vi "Get Test Values.vi"(8 "error in":errorcluster, 11 "Measurements":waveform(dbl)[](array[waveform])) -> (0 "error out":errorcluster, 1 "PWM":T1, 2 "B":T1, 3 "A":T1)   [LabVIEW 2023, in "AI.lvlib"]
uses:
  AI.lvlib
  Test Values.ctl
panel:
  out "subarray 3":dbl[](array[numeric])
  out "subarray 2":dbl[](array[numeric])
  out "subarray":dbl[](array[numeric])
  in  "data":dbl[][](array[numeric]) format="%0.2f"
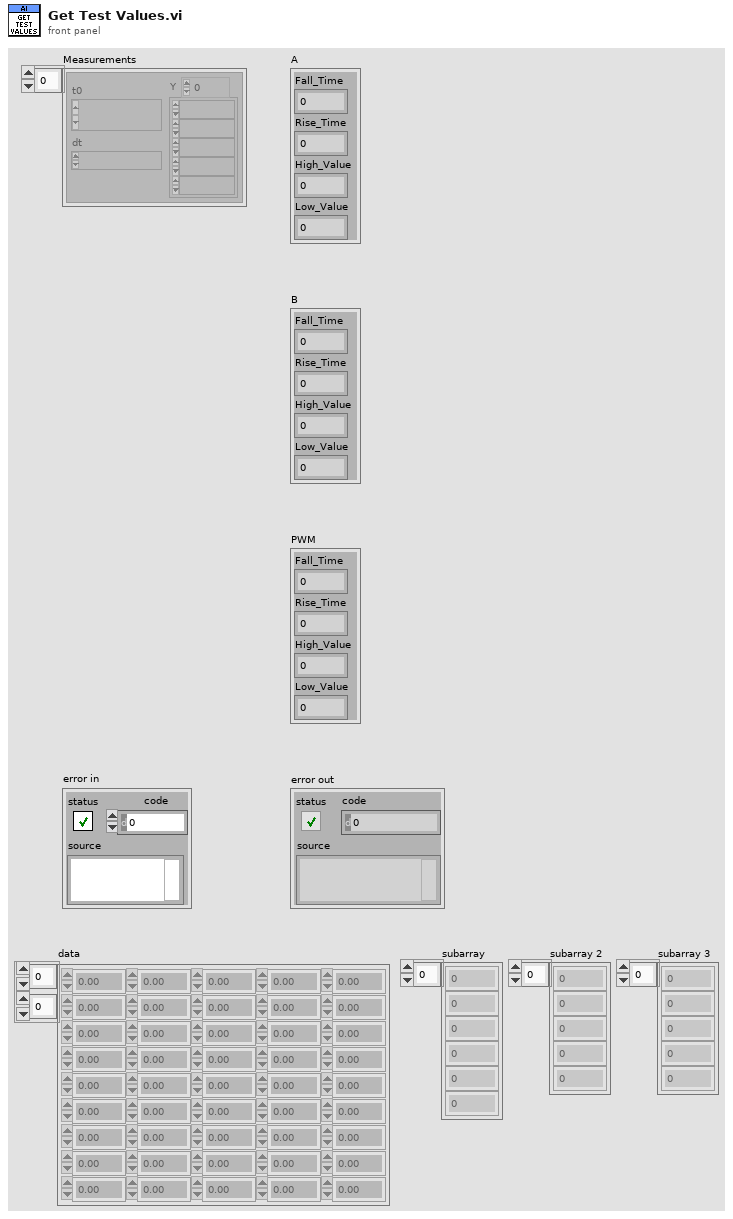
[diagram p1: front panel]
types:
  T1 = typedef "AI.lvlib/Test Values.ctl" = cluster{"Fall_Time":dbl, "Rise_Time":dbl, "High_Value":dbl, "Low_Value":dbl}
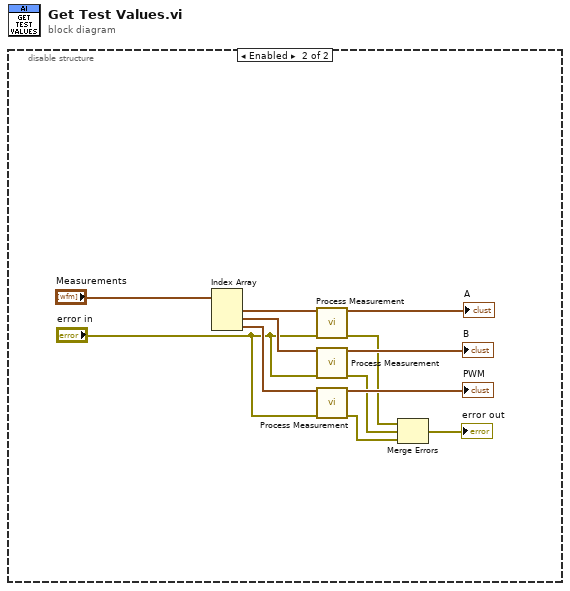
[diagram p0: block diagram]
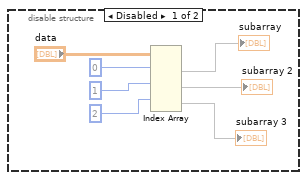
[diagram p2: hidden frame]
diagram:
  n1 = disable-structure shown="Enabled" {
    frame Disabled {
      n2 = Index Array(array="data", index (row) #1=0 ("index (row)"), index (row) #2=1 ("index (row)"), index (row) #3=2 ("index (row)")) -> (element #1=→"subarray":dbl[], element #2=→"subarray 2":dbl[], element #3=→"subarray 3":dbl[])  [unwired: 3 in]
    }
    frame Enabled {
      n3 = Index Array(array="Measurements") -> (element #1=w18:waveform(dbl), element #2=w17:waveform(dbl), element #3=w16:waveform(dbl))  [unwired: 3 in]
      n4 = call "Process Measurement.vi"("Waveform"=w18, "error in"="error in") -> ("Test Values"=→"A":T1, "error out"=w11:errorcluster)  [unwired: 12 in]
      n5 = call "Process Measurement.vi"("Waveform"=w17, "error in"="error in") -> ("Test Values"=→"B":T1, "error out"=w10:errorcluster)  [unwired: 12 in]
      n6 = call "Process Measurement.vi"("Waveform"=w16, "error in"="error in") -> ("Test Values"=→"PWM":T1, "error out"=w9:errorcluster)  [unwired: 12 in]
      n7 = Merge Errors(w11, w10, w9) -> (→"error out":errorcluster)
    }
  }
